vi "Finalization.vi"(8 "error in":errorcluster) -> (0 "error out":errorcluster)   [LabVIEW 2017]
uses:
  ManageMovableObjects/ManRef_mods.ctl
  Display/Display_mods.ctl
  Spaceship/Spaceship_mods.ctl
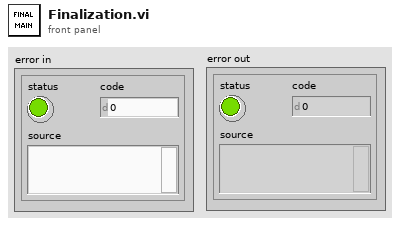
[diagram p1: front panel]
types:
  T1 = typedef "Spaceship_mods.ctl" = enum16{"Init", "Move", "Rotate", "Translate", "GetData", "End"}
  T2 = typedef "Display_mods.ctl" = enum16{"Init", "GetBase", "DrawAster", "DrawShip", "DrawShoot", "Clear", "Close"}
  T3 = typedef "ManRef_mods.ctl" = enum16{"Init", "NewAster", "MoveAll", "DestroyAster", "NewShoot", "DestroyShot", "End"}
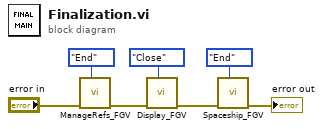
[diagram p0: block diagram]
diagram:
  n1 = call "ManageRefs_FGV.vi"("ManRef_mods"=ManRef_mods."End", "error in"="error in") -> ("error out"=w6:errorcluster)  [unwired: 9 in]
  n2 = call "Display_FGV.vi"("Display_mods"=Display_mods."Close", "error in"=w6) -> ("error out"=w3:errorcluster)  [unwired: 8 in, 1 out]
  n3 = call "Spaceship_FGV.vi"("Spaceship_mods"=Spaceship_mods."End", "error in"=w3) -> ("error out"=→"error out":errorcluster)  [unwired: 8 in, 1 out]
